vi "WritetoCSV.vi"(0 "File path":path, 5 "Array In":string[][](array[string]), 11 "error in":errorcluster) -> (4 "path out":path, 6 "spreadsheet string":string, 15 "error out":errorcluster)   [LabVIEW 2023, in "Unit Testing CA1.lvlib"]
uses:
  Unit Testing CA1.lvlib
panel:
  in  "append to file?":bool
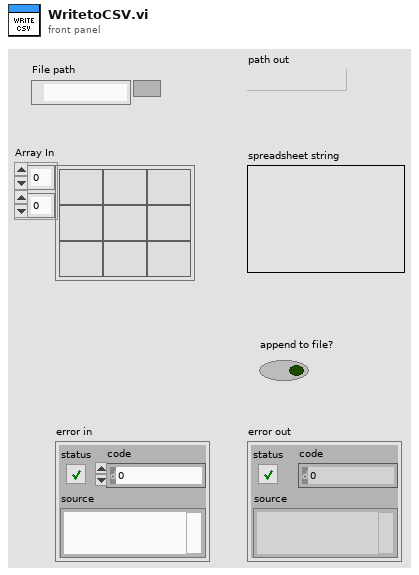
[diagram p1: front panel]
types:
  T1 = enum16{"open", "replace", "create", "open or create", "replace or create", "replace or create with confirmation"}
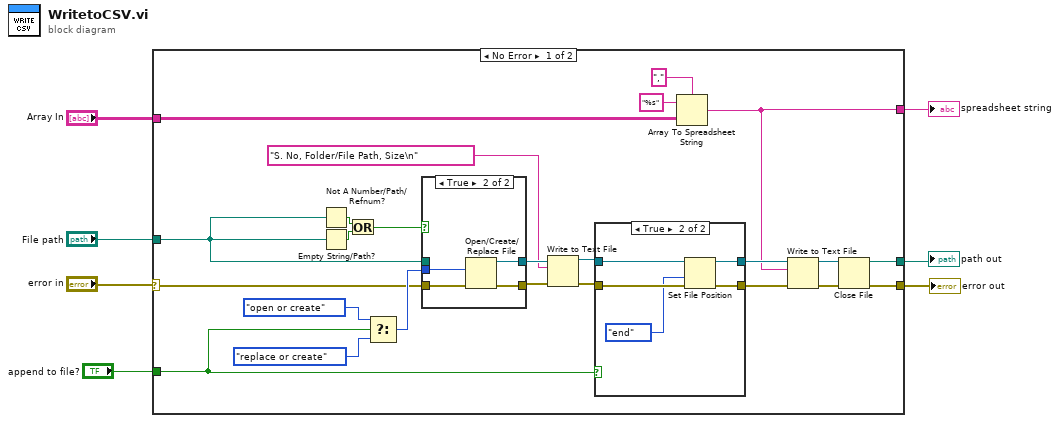
[diagram p0: block diagram]
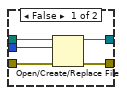
[diagram p3: hidden frame]
diagram:
  n1 = case shown="No Error" "error in" {
    selector: "error in" -> [w20 w48]
    tunnel: [w28 w48] -> w6
    tunnel: "File path" -> [w12 _]
    tunnel: "append to file?" -> [w11 _]
    tunnel: [w10 _] -> w5
    tunnel: [w9 _] -> w4
    tunnel: "Array In" -> [w8 _]
    frame No Error {
      n2 = Not A Number/Path/Refnum?(number/path/refnum=w12) -> (NaN/Path/Refnum?=w23:bool)
      n3 = Empty String/Path?(string/path=w12) -> (empty?=w24:bool)
      n4 = Or(x=w23, y=w24) -> (x .or. y?=w22:bool)
      n5 = Select ("function")(t=T1."open or create" ("operation (0:open)"), s=w11, f=T1."replace or create" ("operation (0:open)")) -> (s? t:f=w21:T1)
      n6 = case shown="True" w22 {
        tunnel: w20 -> [w43 w46]
        tunnel: [w42 w47] -> w14
        tunnel: [w41 w45] -> w15
        tunnel: w12 -> [w40 _]
        tunnel: w21 -> [w39 w44]
        frame False {
          n7 = Open/Create/Replace File(file path (use dialog)=w40, error in=w43, operation (0:open)=w39) -> (refnum out=w41:refnum<file>, error out=w42:errorcluster)  [unwired: 3 in, 1 out]
        }
        frame True {
          n8 = Open/Create/Replace File(error in=w46, operation (0:open)=w44) -> (refnum out=w45:refnum<file>, error out=w47:errorcluster)  [unwired: 4 in, 1 out]
        }
      }
      n9 = Write to Text File(file (use dialog)=w15, text="S. No, Folder/File Path, Size\n", error in=w14) -> (refnum out=w17:refnum<file>, error out=w16:errorcluster)  [unwired: 1 in, 1 out]
      n10 = case shown="True" w11 {
        tunnel: w16 -> [w32 w38]
        tunnel: [w32 w37] -> w19
        tunnel: w17 -> [w33 w35]
        tunnel: [w33 w36] -> w18
        frame False {
        }
        frame True {
          n11 = Set File Position(refnum=w35, from (0:start)=enum16{"start", "end", "current"}."end", error in=w38) -> (refnum out=w36:refnum<file>, error out=w37:errorcluster)  [unwired: 1 in]
        }
      }
      n12 = Array To Spreadsheet String(delimiter (Tab)=",", array=w8, 3:"%s" ("format string")) -> (spreadsheet string=w9:string)
      n13 = Write to Text File(file (use dialog)=w18, text=w9, error in=w19) -> (refnum out=w30:refnum<file>, error out=w29:errorcluster)  [unwired: 1 in, 1 out]
      n14 = Close File(refnum=w30, error in=w29) -> (path=w10:path, error out=w28:errorcluster)
    }
    frame Error {
    }
  }
  "error out" <- w6
  "path out" <- w5
  "spreadsheet string" <- w4
